vi "Set Custom Device Properties.vi"   [LabVIEW 2015, in "J1939 System Definition API Support.lvlib"]
uses:
  J1939 System Definition API Support.lvlib
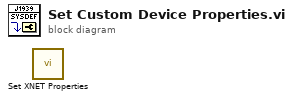
[diagram p0: block diagram]
diagram:
  n1 = call "Set XNET Properties.vi"() -> ()  [unwired: 10 in, 2 out]
